vi "Save ROI Setup Files.vi"(8 "Error In":errorcluster, 10 "ROI_Information_Cluster":T2 {"Norm. XYZ Coordinates"."ROI group ID" format="%#_6f"; "Norm. XYZ Coordinates"."Laser Power (%)" format="%#_6f"; "Norm. XYZ Coordinates"."Zoom" format="%#_6f"; "Norm. XYZ Coordinates"."Frame Size" format="%#_6f"; "Norm. XYZ Coordinates"."Number of lines" format="%#_6f"; "Norm. XYZ Coordinates"."Composite ID" format="%#_6f"; "Norm. XYZ Coordinates"."Angle (deg)" format="%#_6f"; "Norm. XYZ Coordinates"."ROI Time (ns)" format="%#_6f"; "Norm. XYZ Coordinates"."ROI ID" format="%#_6f"; "Norm. XYZ Coordinates"."Pixels in ROI" format="%#_6f"; "Norm. XYZ Coordinates"."ROI index" format="%#_6f"; "Norm. XYZ Coordinates"."Z stop" format="%#_6f"; "Norm. XYZ Coordinates"."Y stop" format="%#_6f"; "Norm. XYZ Coordinates"."X stop" format="%#_6f"; "Norm. XYZ Coordinates"."Z start" format="%#_6f"; "Norm. XYZ Coordinates"."X start" format="%#_6f"; "Norm. XYZ Coordinates"."Y start" format="%#_6f"; "XYZ Coordinates"."ROI group ID" format="%#_6f"; "XYZ Coordinates"."Laser Power (%)" format="%#_6f"; "XYZ Coordinates"."Zoom" format="%#_6f"; "XYZ Coordinates"."Frame Size" format="%#_6f"; "XYZ Coordinates"."Number of lines" format="%#_6f"; "XYZ Coordinates"."Composite ID" format="%#_6f"; "XYZ Coordinates"."Angle (deg)" format="%#_6f"; "XYZ Coordinates"."ROI Time (ns)" format="%#_6f"; "XYZ Coordinates"."ROI ID" format="%#_6f"; "XYZ Coordinates"."Pixels in ROI" format="%#_6f"; "XYZ Coordinates"."ROI index" format="%#_6f"; "XYZ Coordinates"."Z stop" format="%#_6f"; "XYZ Coordinates"."Y stop" format="%#_6f"; "XYZ Coordinates"."X stop" format="%#_6f"; "XYZ Coordinates"."Z start" format="%#_6f"; "XYZ Coordinates"."X start" format="%#_6f"; "XYZ Coordinates"."Y start" format="%#_6f"}, 11 "Experiment data folder path":path) -> (0 "Error Out":errorcluster)   [LabVIEW 2017]
uses:
  Visualisation/Functional Imaging Viewer/Typedefs/ROI parameters data type.ctl
panel:
  out "[Z norm]":dbl[](array[numeric]) format="%#_9g"
  out "Z start":dbl format="%#_10g"
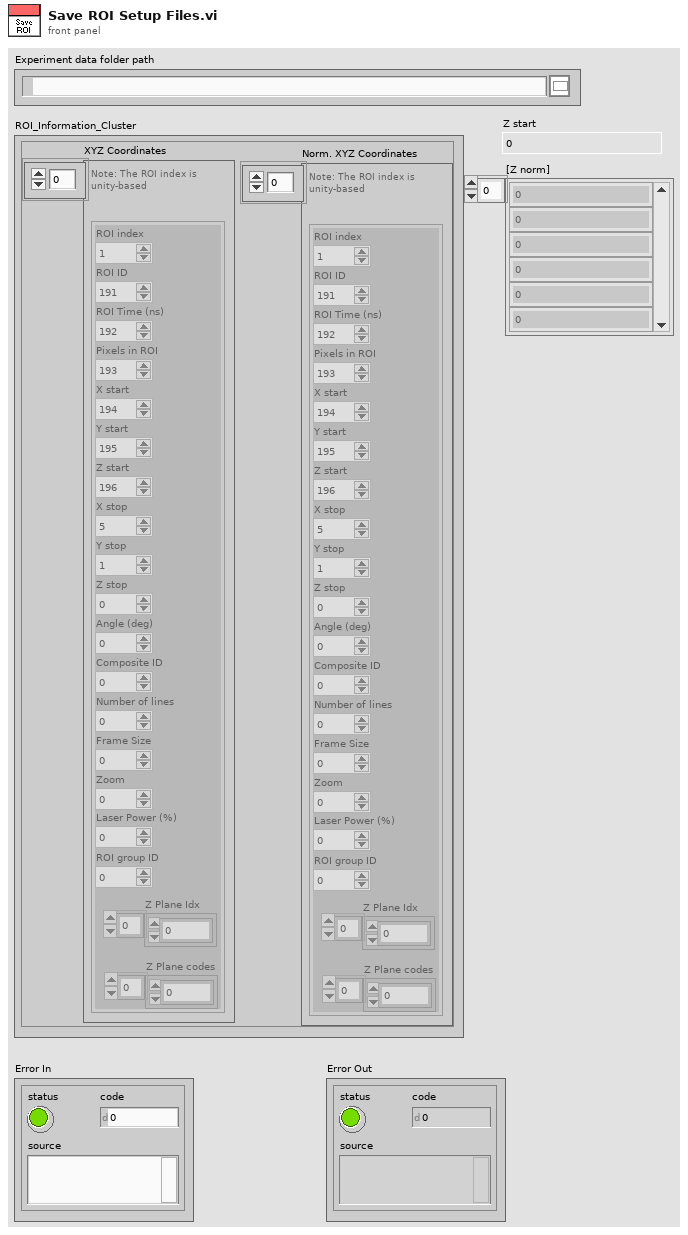
[diagram p1: front panel]
types:
  T1 = typedef "ROI parameters data type.ctl" = cluster{"ROI index":dbl, "ROI ID":dbl, "ROI Time (ns)":dbl, "Pixels in ROI":dbl, "X start":dbl, "Y start":dbl, "Z start":dbl, "X stop":dbl, "Y stop":dbl, "Z stop":dbl, "Angle (deg)":dbl, "Composite ID":dbl, "Number of lines":dbl, "Frame Size":dbl, "Zoom":dbl, "Laser Power (%)":dbl, "ROI group ID":dbl, "Z Plane Idx":i32[], "Z Plane codes":i32[]}
  T2 = cluster{"XYZ Coordinates":T1[], "Norm. XYZ Coordinates":T1[]}
  T3 = typedef "Fixed strings.ctl" = cluster{"ROI file name":string, "Normalised ROI file name":string, "Zplane Pockels values file name":string, "Functional data folder name":string, "Experiment Header file name":string, "Z-stack images folder name":string, "Groups setup rel. path":string, "Groups text file rel. path":string, "TDMS files folder name (F.img)":string, "TDMS files folder name (V.acq)":string, "TDMS files folder name (Pl.acq)":string, "Cycle rel times sequence file":string, "Dynamically called VIs folder name":string, "Time Series folder base name":string}
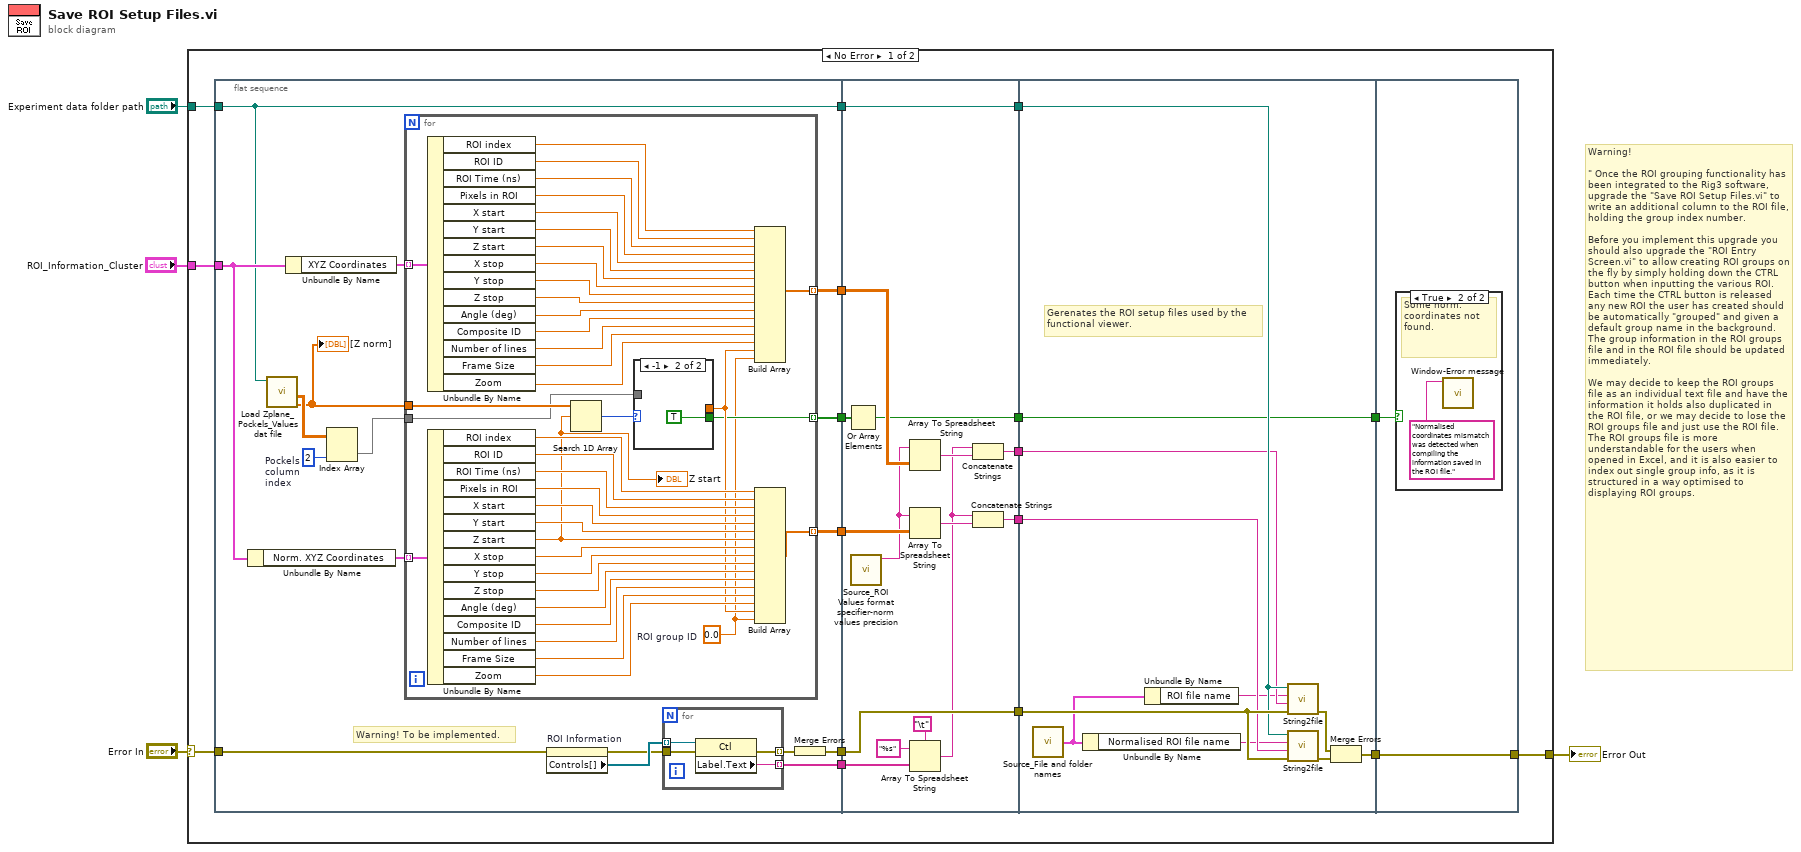
[diagram p0: block diagram]
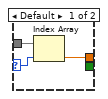
[diagram p2: hidden frame]
diagram:
  # "Warning!\n\n\"\tOnce the ROI grouping functionality has been integrated to the Rig3 software, upgrade the \"Save ROI Setup Files.vi\" to write an additional column to the ROI file, holding the group index number.\n\nBefore you implement this upgrade you should also upgrade the \"ROI Entry Screen.vi\" to allow creating ROI groups on the fly by simply holding down the CTRL button when inputting the various ROI. Each time the CTRL button is released any new ROI the user has created should be automatically \"grouped\" and given a default group name in the background. The group information in the ROI groups file and in the ROI file should be updated immediately.\n\nWe may decide to keep the ROI groups file as an individual text file and have the information it holds also duplicated in the ROI file, or we may decide to lose the ROI groups file and just use the ROI file. The ROI groups file is more understandable for the users when opened in Excel, and it is also easier to index out single group info, as it is structured in a way optimised to displaying ROI groups."
  n1 = case shown="No Error" "Error In" {
    selector: "Error In" -> [w21 w116]
    tunnel: [w14 w116] -> w3
    tunnel: "ROI_Information_Cluster" -> [w12 _]
    tunnel: "Experiment data folder path" -> [w9 _]
    frame No Error {
      n2 = flat-sequence {
        tunnel: w21 -> [w33]
        tunnel: [w22] -> w20
        tunnel: [w36] -> w19
        tunnel: [w35] -> w18
        tunnel: [w31] -> w17
        tunnel: w12 -> [w30]
        tunnel: [w26] -> w10
        tunnel: w9 -> [w26]
        tunnel: [w23] -> w8
        tunnel: w20 -> [w99]
        tunnel: w19 -> [w98]
        tunnel: w18 -> [w96]
        tunnel: w17 -> [w97]
        tunnel: [w97] -> w16
        tunnel: [w93] -> w15
        tunnel: [w92] -> w13
        tunnel: [w90] -> w11
        tunnel: w10 -> [w90]
        tunnel: w8 -> [w88]
        tunnel: [w87] -> w5
        tunnel: w16 -> [w112]
        tunnel: w15 -> [w109]
        tunnel: w13 -> [w108]
        tunnel: w11 -> [w110]
        tunnel: [w111] -> w7
        tunnel: [w102] -> w6
        tunnel: w5 -> [w102]
        tunnel: [w114] -> w14
        tunnel: w7 -> [w114]
        tunnel: w6 -> [w113]
        frame #0 {
          w28 = 2  # Pockels column index
          # "Warning! To be implemented."
          n3 = Unbundle By Name(w30) -> ("Norm. XYZ Coordinates"=w29:T1[])
          n4 = call "Load Zplane_Pockels_Values dat file.vi"("Experiment data folder path"=w26) -> ("[AOL Z (um)]"=w24:dbl[], "Zplane_Pockels_Values file data (header removed)"=w27:dbl[][])  [unwired: 5 in, 4 out]
          "[Z norm]" <- w24
          n5 = Unbundle By Name(w30) -> ("XYZ Coordinates"=w37:T1[])
          n6 = Index Array(array=w27, index (col)=w28) -> (element=w25:dbl[])  [unwired: 1 in]
          n7 = for {
            tunnel: w37 -> [w78] mode=indexing
            tunnel: w29 -> [w61] mode=indexing
            tunnel: [w60] -> w36 mode=indexing
            tunnel: [w59] -> w35 mode=indexing
            tunnel: w25 -> [w42]
            tunnel: w24 -> [w44]
            tunnel: [w40] -> w23 mode=indexing
            w39 = 0.0  # ROI group ID
            n8 = Unbundle By Name(w78) -> ("ROI index"=w77:dbl, "ROI ID"=w76:dbl, "ROI Time (ns)"=w75:dbl, "Pixels in ROI"=w74:dbl, "X start"=w73:dbl, "Y start"=w72:dbl, "Z start"=w71:dbl, "X stop"=w70:dbl, "Y stop"=w69:dbl, "Z stop"=w56:dbl, "Angle (deg)"=w57:dbl, "Composite ID"=w55:dbl, "Number of lines"=w54:dbl, "Frame Size"=w53:dbl, "Zoom"=w52:dbl)
            n9 = Unbundle By Name(w61) -> ("ROI index"=w62:dbl, "ROI ID"=w63:dbl, "ROI Time (ns)"=w64:dbl, "Pixels in ROI"=w65:dbl, "X start"=w66:dbl, "Y start"=w46:dbl, "Z start"=w45:dbl, "X stop"=w47:dbl, "Y stop"=w67:dbl, "Z stop"=w68:dbl, "Angle (deg)"=w58:dbl, "Composite ID"=w51:dbl, "Number of lines"=w50:dbl, "Frame Size"=w49:dbl, "Zoom"=w48:dbl)
            "Z start" <- w45
            n10 = Search 1D Array(1D array=w44, element=w45) -> (index of element=w43:i32)  [unwired: 1 in]
            n11 = case shown="-1" w43 {
              selector: w43 -> [w80 _]
              tunnel: [_ TRUE] -> w40
              tunnel: w42 -> [w81 _]
              tunnel: [w79 _] -> w41
              frame Default {
                n12 = Index Array(array=w81, index=w80) -> (element=w79:dbl)
              }
              frame -1 {
              }
            }
            n13 = Build Array(w77, w76, w75, w74, w73, w72, w71, w70, w69, w56, w57, w55, w54, w53, w52, w41, w39) -> (w60:dbl[])
            n14 = Build Array(w62, w63, w64, w65, w66, w46, w45, w47, w67, w68, w58, w51, w50, w49, w48, w41, w39) -> (w59:dbl[])
          }
          n15 = property on="ROI Information" class="Clust (strict)"(error in=w33) -> (error out=w34:errorcluster, "Controls[]"=w38:refnum<vi>[])  [unwired: 1 in, 1 out]
          n16 = for {
            tunnel: w38 -> [w86] mode=indexing
            tunnel: [w85] -> w22 mode=indexing
            tunnel: [w84] -> w32 mode=indexing
            tunnel: w34 -> [w83]
            n17 = property class="Ctl"(reference=w86, error in=w83) -> (error out=w84:errorcluster, "Label.Text"=w85:string)  [unwired: 1 out]
          }
          n18 = Merge Errors(w32) -> (w31:errorcluster)
        }
        frame #1 {
          n19 = Or Array Elements(Boolean array=w88) -> (logical OR=w87:bool)
          n20 = call "Source_ROI Values format specifier-norm values precision.vi"() -> ("format (%.3f)"=w89:string)  [unwired: 11 in]
          n21 = Array To Spreadsheet String(array=w98, 3:w89) -> (spreadsheet string=w94:string)  [unwired: 1 in]
          n22 = Array To Spreadsheet String(array=w96, 3:w89) -> (spreadsheet string=w95:string)  [unwired: 1 in]
          n23 = Array To Spreadsheet String(delimiter (Tab)="\t", array=w99, 3:"%s" ("format string")) -> (spreadsheet string=w91:string)
          n24 = Concatenate Strings(w91, w94) -> (w93:string)
          n25 = Concatenate Strings(w91, w95) -> (w92:string)
        }
        frame #2 {
          # "Gerenates the ROI setup files used by the\nfunctional viewer."
          n26 = call "Source_File and folder names.vi"() -> ("Fixed strings"=w105:T3)  [unwired: 1 in]
          n27 = Unbundle By Name(w105) -> ("Normalised ROI file name"=w106:string)
          n28 = Unbundle By Name(w105) -> ("ROI file name"=w107:string)
          n29 = call "String2file.vi"("Error In"=w112, "Input String"=w109, "FileName"=w107, "Base Path"=w110) -> ("Error Out"=w104:errorcluster)  [unwired: 7 in]
          n30 = call "String2file.vi"("Error In"=w112, "Input String"=w108, "FileName"=w106, "Base Path"=w110) -> ("Error Out"=w103:errorcluster)  [unwired: 7 in]
          n31 = Merge Errors(w104, w103) -> (w111:errorcluster)
        }
        frame #3 {
          n32 = case shown="True" w113 {
            frame False {
            }
            frame True {
              # "Some norm. coordinates not found."
              n33 = call "Window-Error message.vi"("Message"="Normalised coordinates mismatch was detected when compiling the information saved in the ROI file." ("Error Source")) -> ()  [unwired: 10 in, 1 out]
            }
          }
        }
      }
    }
    frame Error {
    }
  }
  "Error Out" <- w3
